vi "Configure Data Clock.vi"(6 "External Reference Frequency (13 MHz)":dbl=13000000.0, 7 "External Data Clock (0: Normal)":u16(ring) items=["Normal", "Symbol"], 8 "error in (no error)":errorcluster, 9 "Reference Source (0: Internal)":u16(ring) items=["Internal", "External"], 10 "Data Clock Source (0: Internal)":u16(ring) items=["Internal", "External"], 11 "VISA resource name":refnum<visa-resource-name>) -> (0 "error out":errorcluster, 3 "VISA resource name out":refnum<visa-resource-name>)   [LabVIEW 2011, in "Agilent PSG MXG Series.lvlib"]
doc: "Configures the data clock and the bit-clock.\n\n<B>Notes:</B>\n(1) This VI is valid only in E8267C, E8267D.\n\n(2) For E8267C, this VI is valid only when the instrument installs <B>Option 002</B> (Internal baseband generator) or <B>Option 602</B> (Digital bus baseband generator).\n\n(3) For E8267D, this VI is valid only when the instrument installs <B>Option 601</B> or <B>Option 602</B> (Internal baseband generator)."
uses:
  Agilent PSG MXG Series.lvlib
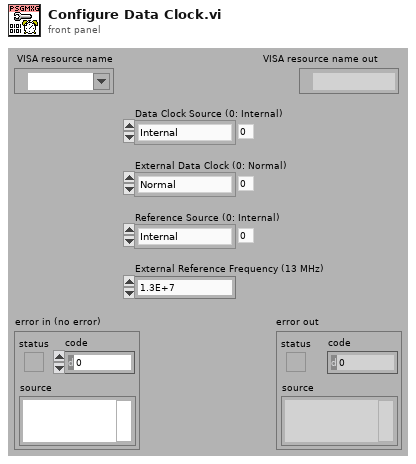
[diagram p1: front panel]
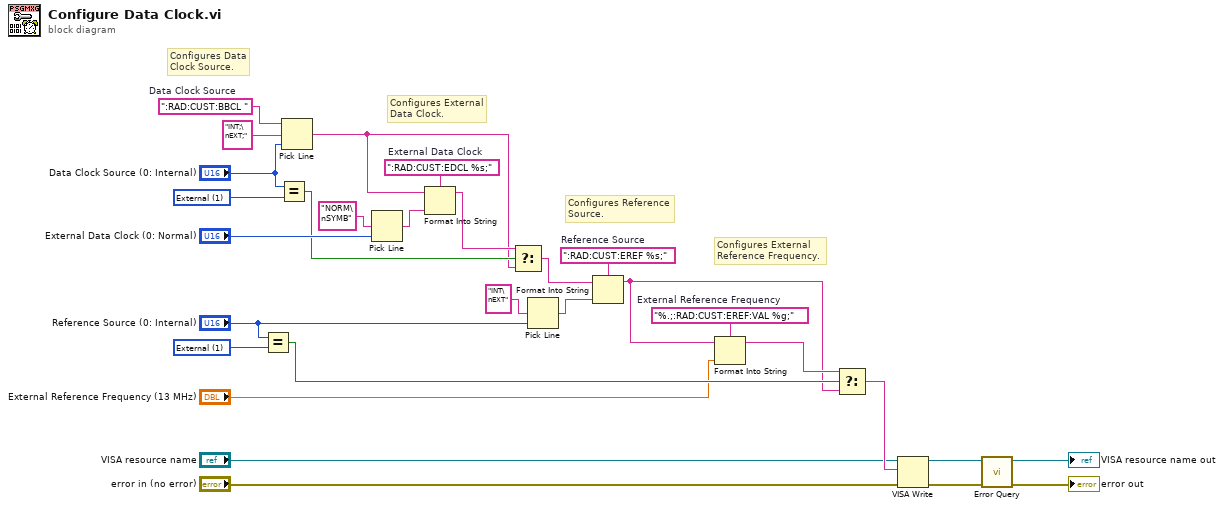
[diagram p0: block diagram]
diagram:
  w13 = u16 1 items=["Internal", "External"] ("Data Clock Source (0: Internal)")
  w7 = ":RAD:CUST:EREF %s;"  # Reference Source
  w21 = u16 1 items=["Internal", "External"] ("Reference Source (0: Internal)")
  w23 = "%.;:RAD:CUST:EREF:VAL %g;"  # External Reference Frequency
  w27 = ":RAD:CUST:EDCL %s;"  # External Data Clock
  w29 = ":RAD:CUST:BBCL "  # Data Clock Source
  # "Configures External\nReference Frequency."
  # "Configures Reference\nSource."
  # "Configures External\nData Clock."
  # "Configures Data\nClock Source."
  n1 = Equal?(x="Reference Source (0: Internal)", y=w21) -> (x = y?=w20:bool)
  n2 = Equal?(x="Data Clock Source (0: Internal)", y=w13) -> (x = y?=w12:bool)
  n3 = Pick Line(string ("")=w29, multi-line string="INT;\nEXT;", line index="Data Clock Source (0: Internal)") -> (output string=w10:string)
  n4 = Pick Line(multi-line string="NORM\nSYMB", line index="External Data Clock (0: Normal)") -> (output string=w9:string)  [unwired: 1 in]
  n5 = Format Into String(format string=w27, initial string=w10, w9) -> (resulting string=w11:string)  [unwired: 1 in, 1 out]
  n6 = Select(t=w11, s=w12, f=w10) -> (s? t:f=w8:string)
  n7 = Pick Line(multi-line string="INT\nEXT", line index="Reference Source (0: Internal)") -> (output string=w6:string)  [unwired: 1 in]
  n8 = Format Into String(format string=w7, initial string=w8, w6) -> (resulting string=w5:string)  [unwired: 1 in, 1 out]
  n9 = Format Into String(format string=w23, initial string=w5, "External Reference Frequency (13 MHz)") -> (resulting string=w19:string)  [unwired: 1 in, 1 out]
  n10 = Select(t=w19, s=w20, f=w5) -> (s? t:f=w17:string)
  n11 = VISA Write(VISA resource name="VISA resource name", write buffer=w17, error in (no error)="error in (no error)") -> (VISA resource name out=w16:refnum<visa-resource-name>, error out=w15:errorcluster)  [unwired: 1 out]
  n12 = call "Error Query.vi"("error in (no error)"=w15, "VISA resource name"=w16) -> ("error out"=→"error out":errorcluster, "VISA resource name out"=→"VISA resource name out":refnum<visa-resource-name>)  [unwired: 6 in, 2 out]
